vi "speedSet.vi"(8 "error in (no error)":errorcluster, 11 "VISA resource name":refnum<visa-resource-name>="ASRL6::INSTR") -> (0 "error out (no error)":errorcluster, 1 "spm":string="0", 2 "rpm":string="0", 3 "speed":string="0.0", 4 "RPM":dbl(knob) scale=0.0..200.0, 5 "SPEED":dbl(knob) scale=0.0..50.0, 6 "SPM":dbl(knob) scale=0.0..200.0, 7 "Running":bool)   [LabVIEW 2018]
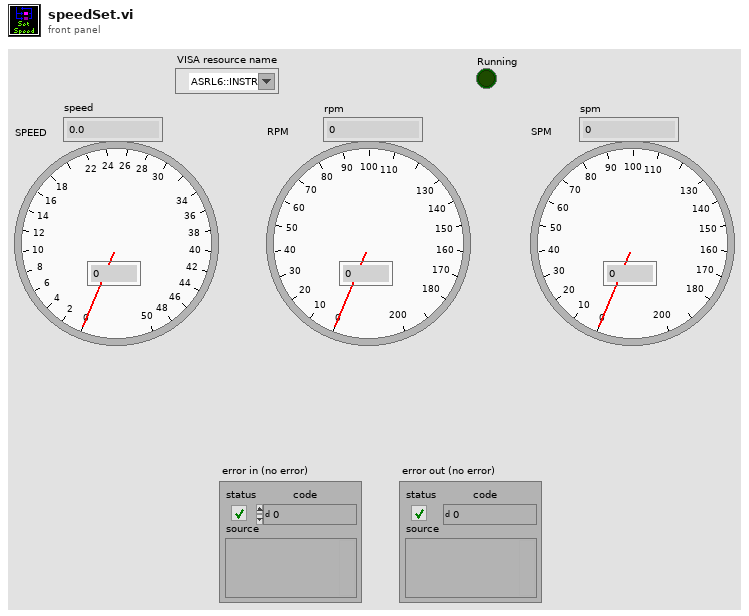
[diagram p1: front panel]
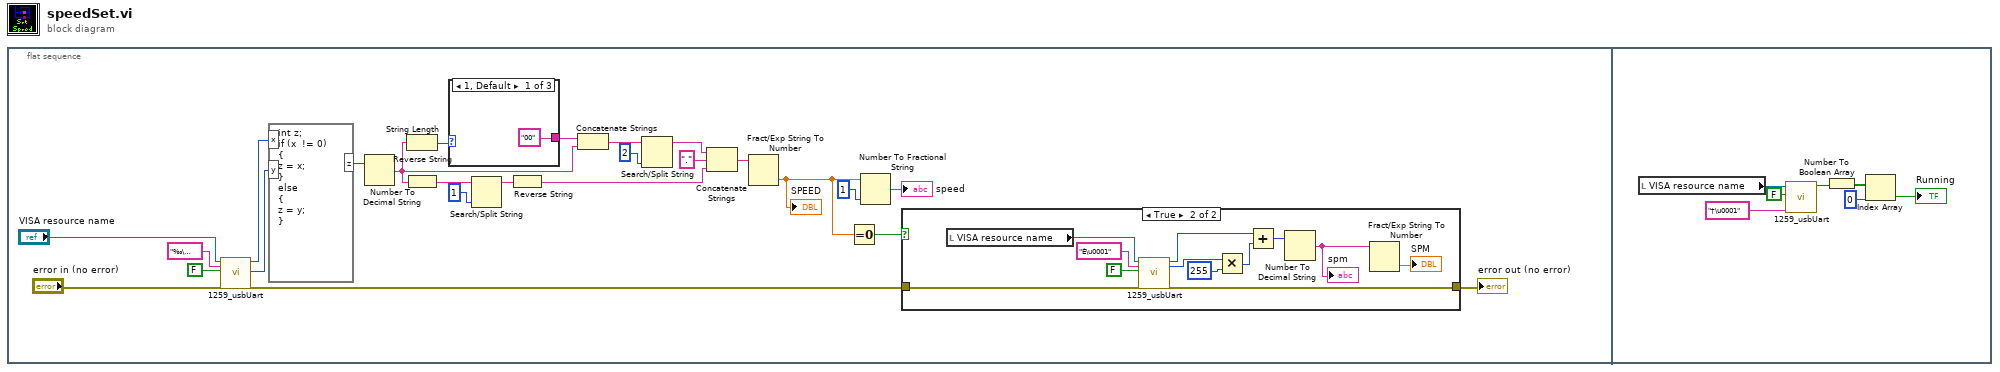
[diagram p0: block diagram]
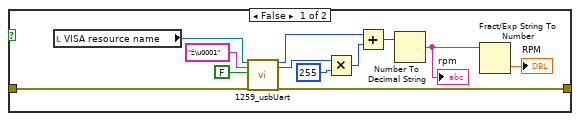
[diagram p2: hidden frame]
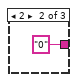
[diagram p3: hidden frame]
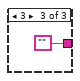
[diagram p4: hidden frame]
diagram:
  n1 = flat-sequence {
    frame #0 {
      n2 = call "1259_usbUart.vi"("VISA resource name"="VISA resource name", "write buffer"="‰\u0004", "sdFeature"=FALSE, "error in (no error)"="error in (no error)") -> ("number[0]"=w22:u32, "number[2]"=w8:u32, "error out"=w3:errorcluster)  [unwired: 13 out]
      n3 = formula code="int z;\nif (x  != 0)\n{\nz = x;\n}\nelse\n{\nz = y;\n}"("x"=w22, "y"=w8) -> ("z"=w23:i32)
      n4 = Number To Decimal String(number=w23) -> (decimal integer string=w11:string)  [unwired: 1 in]
      n5 = String Length(string=w11) -> (length=w13:i32)
      n6 = Reverse String(1:w11) -> (0:w21:string)
      n7 = case shown="1, Default" w13 {
        tunnel: ["00" "0" ""] -> w12
        frame 1, Default {
        }
        frame 2 {
        }
        frame 3 {
        }
      }
      n8 = Search/Split String(string=w21, offset (0)=1) -> (substring before match=w20:string)  [unwired: 1 in, 2 out]
      n9 = Reverse String(1:w20) -> (0:w18:string)
      n10 = Concatenate Strings(w12, w11) -> (w10:string)
      n11 = Search/Split String(string=w10, offset (0)=2) -> (substring before match=w19:string)  [unwired: 1 in, 2 out]
      n12 = Concatenate Strings(w19, "." ("string"), w18) -> (w9:string)
      n13 = Fract/Exp String To Number(string=w9) -> (number=w4:dbl)  [unwired: 3 in, 1 out]
      "SPEED" <- w4
      n14 = Equal To 0?(x=w4) -> (x = 0?=w1:bool)
      n15 = Number To Fractional String(number=w4, precision (6)=i16 1) -> (F-format string=→"speed":string)  [unwired: 2 in]
      n16 = case shown="True" w1 {
        tunnel: w3 -> [w27 w41]
        tunnel: [w26 w40] -> w2
        frame False {
          n17 = local read "VISA resource name"() -> (w37:refnum<visa-resource-name>)
          n18 = call "1259_usbUart.vi"("VISA resource name"=w37, "write buffer"="ž\u0001", "sdFeature"=FALSE, "error in (no error)"=w27) -> ("number[0]"=w34:u32, "number[1]"=w36:u32, "error out"=w26:errorcluster)  [unwired: 13 out]
          n19 = Multiply(x=w36, y=u32 255) -> (x*y=w35:u32)
          n20 = Add(x=w34, y=w35) -> (x+y=w33:u32)
          n21 = Number To Decimal String(number=w33) -> (decimal integer string=w31:string)  [unwired: 1 in]
          "rpm" <- w31
          n22 = Fract/Exp String To Number(string=w31) -> (number=→"RPM":dbl)  [unwired: 3 in, 1 out]
        }
        frame True {
          n23 = local read "VISA resource name"() -> (w45:refnum<visa-resource-name>)
          n24 = call "1259_usbUart.vi"("VISA resource name"=w45, "write buffer"="È\u0001", "sdFeature"=FALSE, "error in (no error)"=w41) -> ("number[0]"=w48:u32, "number[1]"=w46:u32, "error out"=w40:errorcluster)  [unwired: 13 out]
          n25 = Multiply(x=w46, y=u32 255) -> (x*y=w47:u32)
          n26 = Add(x=w48, y=w47) -> (x+y=w49:u32)
          n27 = Number To Decimal String(number=w49) -> (decimal integer string=w39:string)  [unwired: 1 in]
          "spm" <- w39
          n28 = Fract/Exp String To Number(string=w39) -> (number=→"SPM":dbl)  [unwired: 3 in, 1 out]
        }
      }
      "error out (no error)" <- w2
    }
    frame #1 {
      n29 = local read "VISA resource name"() -> (w59:refnum<visa-resource-name>)
      n30 = call "1259_usbUart.vi"("VISA resource name"=w59, "write buffer"="†\u0001", "sdFeature"=FALSE) -> ("number[0]"=w56:u32)  [unwired: 1 in, 15 out]
      n31 = Number To Boolean Array(number=w56) -> (Boolean array=w55:bool[])
      n32 = Index Array(array=w55, index=0) -> (element=→"Running":bool)
    }
  }
